vi "Lookup PluginGUI Tasks.vi"(8 "error in (no error)":errorcluster, 11 "GUI Manager Module in":refnum<class "GUI Manager Module.lvclass">) -> (0 "error out":errorcluster, 3 "GUI Manager Module out":refnum<class "GUI Manager Module.lvclass">)   [LabVIEW 2020, in "VolatusGUI.lvlib" / "GUI Manager Module.lvclass"]
uses:
  GUI Manager Module.lvclass
  C:/dev/lv20CE/relink/lv-volatus/Volatus/Module/Module.lvclass
  VolatusConfig/Meta Name.ctl
  PluginGUI/PluginGUI.lvclass
  Volatus/Module/Module.lvclass
  GUI Manager Module.lvclass/GUI Manager Module.ctl
  Volatus/Module/Module.lvclass/Module.ctl
  Volatus/VolatusAPI/VolatusAPI.lvclass/VolatusAPI.ctl
  VolatusConfig/VolatusConfigElement/VolatusConfigElement.lvclass/VolatusConfigElement.ctl
  Plugin Info.ctl
  VolatusConfig/VolatusConfigElement/Element.vi
  VolatusConfig/Node/Node Config.lvclass
  C:/dev/lv20CE/relink/lv-volatus/VolatusConfig/VolatusConfigElement/VolatusConfigElement.lvclass
  lv-cdm/CDM-Config/Config Lookup/Match Meta.vi
  lv-cdm/CDM-Config/Config Element/Owner.vi
  lv-cdm/CDM-Config/Config Manager/Lookup Descendant.vi
  lv-cdm/CDM-Config/Config Filter/Config Lookup.lvclass
  Volatus/VolatusAPI/VolatusAPI.lvclass
  VolatusConfig/VolatusConfig.lvlib
  VolatusConfig/VolatusConfigElement/VolatusConfigElement.lvclass
  lv-cdm/CDM-Config/Config Element/Config Element.lvclass
  C:/dev/lv20CE/relink/lv-volatus/VolatusGUI/GUI Manager Module/GUI Manager Module.lvclass
  C:/dev/lv20CE/relink/lv-volatus/VolatusGUI/PluginGUI/PluginGUI.lvclass
  C:/dev/lv20CE/relink/lv-volatus/VolatusConfig/Node/Node Config.lvclass
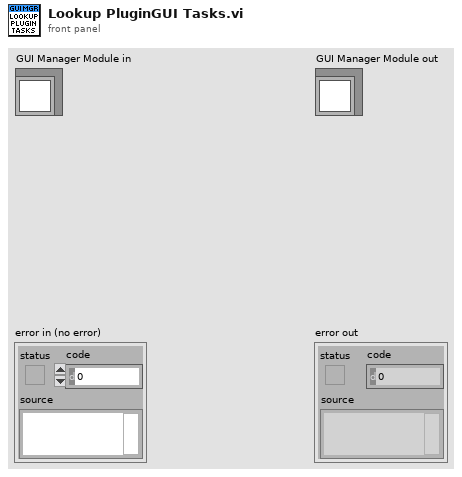
[diagram p1: front panel]
types:
  T1 = typedef "VolatusConfig.lvlib/Meta Name.ctl" = enum16{"VL_Type", "VL_Node_IP", "VL_Node_Type", "VL_Task_Type", "VL_Group_Type", "VL_Channel_Type", "VL_Channel_DataType", "VL_Config_Version", "VL_Overlay_Type", "VL_Config_Hash"}
  T2 = typedef "VolatusGUI.lvlib/GUI Manager Module.lvclass/Plugin Info.ctl" = cluster{"Path":path, "Module ID":string, "Filename":string}
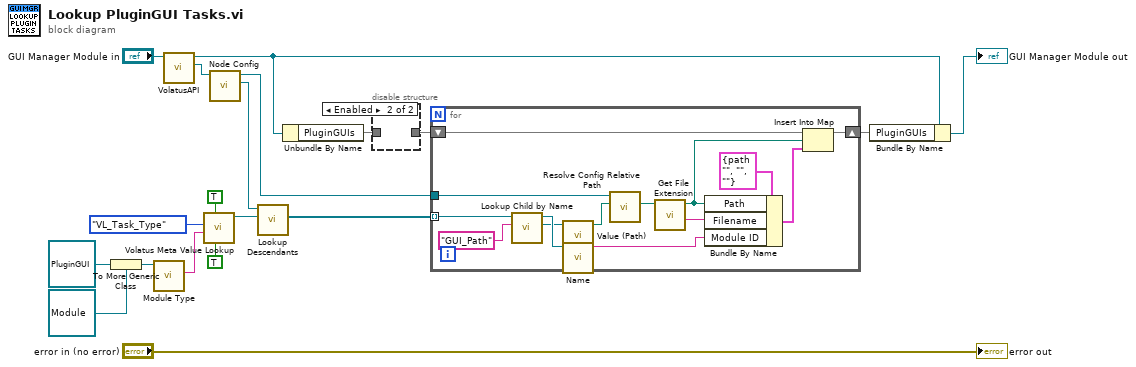
[diagram p0: block diagram]
diagram:
  n1 = To More Generic Class(target class=refnum<class "Module.lvclass"> refnum ("Volatus:Module"), reference=refnum<class "PluginGUI.lvclass"> refnum ("VolatusGUI:PluginGUI.lvclass")) -> (generic class reference=w10:refnum<class "Module.lvclass">)
  n2 = call-dynamic "Module Type.vi"("Module in"=w10) -> ("Module Type"=w16:string)  [unwired: 10 in]
  n3 = call "VolatusAPI.vi"("Module in"="GUI Manager Module in") -> ("VolatusAPI"=w18:refnum<class "VolatusAPI.lvclass">, "Module out"=w6:refnum<class "GUI Manager Module.lvclass">)  [unwired: 9 in]
  n4 = call "Volatus Meta Value Lookup.vi"("Exact Value (F)"=TRUE, "Don't Recurse Past Match (F)"=TRUE, "Value"=w16, "Meta Name"=Meta_Name."VL_Task_Type") -> ("Config Lookup out"=w11:refnum<class "Config Lookup.lvclass">)  [unwired: 6 in, 1 out]
  n5 = call "Node Config.vi"("VolatusAPI in"=w18) -> ("Node Config"=w12:refnum<class "Node Config.lvclass">, "VolatusAPI out"=w7:refnum<class "VolatusAPI.lvclass">)  [unwired: 9 in]
  n6 = call "Lookup Descendants.vi"("Lookup"=w11, "VolatusConfigElement in"=w12) -> ("Descendants"=w8:refnum<class "Config Element.lvclass">[])  [unwired: 7 in, 2 out]
  n7 = Unbundle By Name(w6) -> ("PluginGUIs"=w4:map{path, T2})
  n8 = disable-structure shown="Enabled" {
    disable-tunnel: [w20 _] -> w5
    disable-tunnel: w4 -> [w20 _]
    frame Disabled {
    }
    frame Enabled {
    }
  }
  n9 = for {
    tunnel: w8 -> [w34] mode=indexing
    tunnel: w7 -> [w31]
    shift-right: [w23] -> w2
    shift-left: w5 -> [w24]
    n10 = call "Lookup Child by Name.vi"("Name"="GUI_Path", "Config Element in"=w34) -> ("Child"=w30:refnum<class "Config Element.lvclass">, "Config Element out"=w33:refnum<class "Config Element.lvclass">)  [unwired: 6 in, 2 out]
    n11 = call "Value (Path).vi"("Config Element in"=w30) -> ("Path Value"=w29:path)  [unwired: 9 in, 1 out]
    n12 = call "Name.vi"("Config Element in"=w33) -> ("Name"=w25:string)  [unwired: 9 in, 1 out]
    n13 = call "Resolve Config Relative Path.vi"("Path"=w29, "VolatusAPI in"=w31) -> ("Resolved Path"=w28:path)  [unwired: 7 in, 2 out]
    n14 = call <vilib>:"Get File Extension.vi"("file"=w28) -> ("filename without extension"=w26:string, "dup file"=w21:path)  [unwired: 6 in, 3 out]
    n15 = Bundle By Name(cluster=T2 {"Path"=path "", "Module ID"="", "Filename"=""} ("Plugin Info"), "Path"=w21, "Filename"=w26, "Module ID"=w25) -> (w22:T2)
    n16 = Insert Into Map(map in=w24, key=w21, value=w22) -> (map out=w23:map{path, T2})  [unwired: 2 out]
  }
  n17 = Bundle By Name(cluster=w6, "PluginGUIs"=w2) -> (→"GUI Manager Module out":refnum<class "GUI Manager Module.lvclass">)
  "error out" <- "error in (no error)"
